vi "mosbus主设备.vi"(5 "holding register values":u16[](array[numeric]) caption="保持寄存器值", 7 "starting address":u16 caption="起始地址", 10 "unit ID":u8=1 caption="单元ID", 11 "VISA resource name":refnum<visa-resource-name> caption="VISA资源名称") -> ()   [LabVIEW 2016]
uses:
  <vilib>/Modbus/master/Create Master Instance (Serial).vi
  <vilib>/Modbus/master/Modbus Master.lvclass
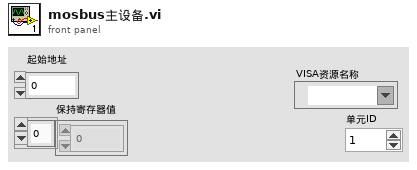
[diagram p1: front panel]
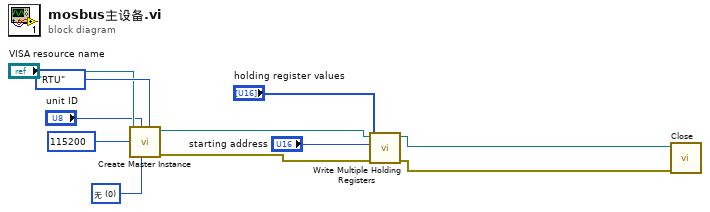
[diagram p0: block diagram]
diagram:
  w5 = u16 0 items=["无", "奇", "偶"] ("parity (Even)")
  n1 = call-poly <vilib>:"Create Master Instance.vi"("serial type"=enum16{"RTU", "ASCII"}."RTU", "parity (Even)"=w5, "unit ID"="unit ID", "baud rate (9600)"=u32 115200, "VISA resource name"="VISA resource name") -> ("error out"=w10:errorcluster, "serial master instance"=w11:refnum<class "Modbus Master.lvclass">)  [unwired: 5 in]
  n2 = call-dynamic "Write Multiple Holding Registers.vi"("error in (no error)"=w10, "holding register values"="holding register values", "starting address"="starting address", "Modbus master in"=w11) -> ("error out"=w8:errorcluster, "Modbus master out"=w9:refnum<class "Modbus Master.lvclass">)  [unwired: 6 in]
  n3 = call-dynamic "Close.vi"("error in (no error)"=w8, "Modbus master in"=w9) -> ()  [unwired: 9 in, 1 out]
